vi "MS Operation.vi"(6 "PID Cluster":T3={"L1 to L4 PID Cluster"={"L1 PID Gains"={"Kp"=0.005, "Kd"=0.5, "Ki"=0.0005}, "L2 PID Gains"={"Kp"=0.01, "Kd"=1.0, "Ki"=0.005}, "L3 PID Gains"={"Kp"=0.05, "Kd"=1.0, "Ki"=0.0005}, "L4 PID Gains"={"Kp"=0.1, "Kd"=0.1, "Ki"=0.0005}}, "Stage PID Cluster"={"Stage Z PID"={"Kp"=0.0005, "Kd"=0.001, "Ki"=0.0}, "Stage Y PID"={"Kp"=0.0003, "Kd"=0.01, "Ki"=0.0}, "Stage X PID"={"Kp"=0.0003, "Kd"=0.01, "Ki"=0.0}}, "OCT Z PID Gains"={"Kp"=0.0003, "Kd"=0.0001, "Ki"=0.01}}, 8 "error in":errorcluster, 9 "Offset Home 2 RCM":dbl[](array[numeric])=[0.0, 0.0, 0.0, 0.0], 10 "Prev Posit Cluster":T2={"Prev L1 to L4 Posit"=[-0.5319, -0.035669172703475985, -2.0566170657346783, 0.9099264705882353], "Prev Stage Posit"=[6.002553885707208, 5.996566124542428, 5.995469940427586], "Prev OCT Z Posit"=-0.0}, 11 "FPGA VI Reference In":refnum<k20>) -> (0 "error out":errorcluster, 2 "Last Posit Cluster":T1={"Last L1 to L4 Posit"=[0.0, 0.0, 0.0, 0.0], "Last Stage Posit"=[6.0, 6.0, 6.0], "Last OCT Z Posit"=0.0}, 3 "FPGA VI Reference Out":refnum<k20>)   [LabVIEW 2016]
uses:
  Global Variables.vi
  <vilib>/Platform/TimedLoop/XDataNode/wakeup.ctl
  <vilib>/Platform/TimedLoop/XDataNode/XDNodeRunTimeDep.lvlib
  <vilib>/Platform/TimedLoop/XDataNode/nitl_modes.ctl
  <vilib>/Platform/TimedLoop/XDataNode/timing_clust.ctl
  <vilib>/platform/TimedLoop/XDataNode/XDataNode.xnode
  <vilib>/rvi/interface/nirviReadWriteControl/nirviReadWriteControl.xnode
  Library/KevinLibraryAll/labview/KevLib01.lvlib
  FPGA Bitfiles/PhantomControlPI_FPGATarget_QuadCtr2_E2412E44.lvbitx
  IRISS_FPGA_IO.vi
  NiFpgaLv.dll
  <vilib>/Utility/error.llb/Error Cluster From Error Code.vi
  <vilib>/rvi/errors/niLvFpgaAdjustHostInterfaceError.vi
panel:
  out "Accurus Remote cmd":T4
  out "L1 to L4 Remote cmd":sgl[](array[numeric])
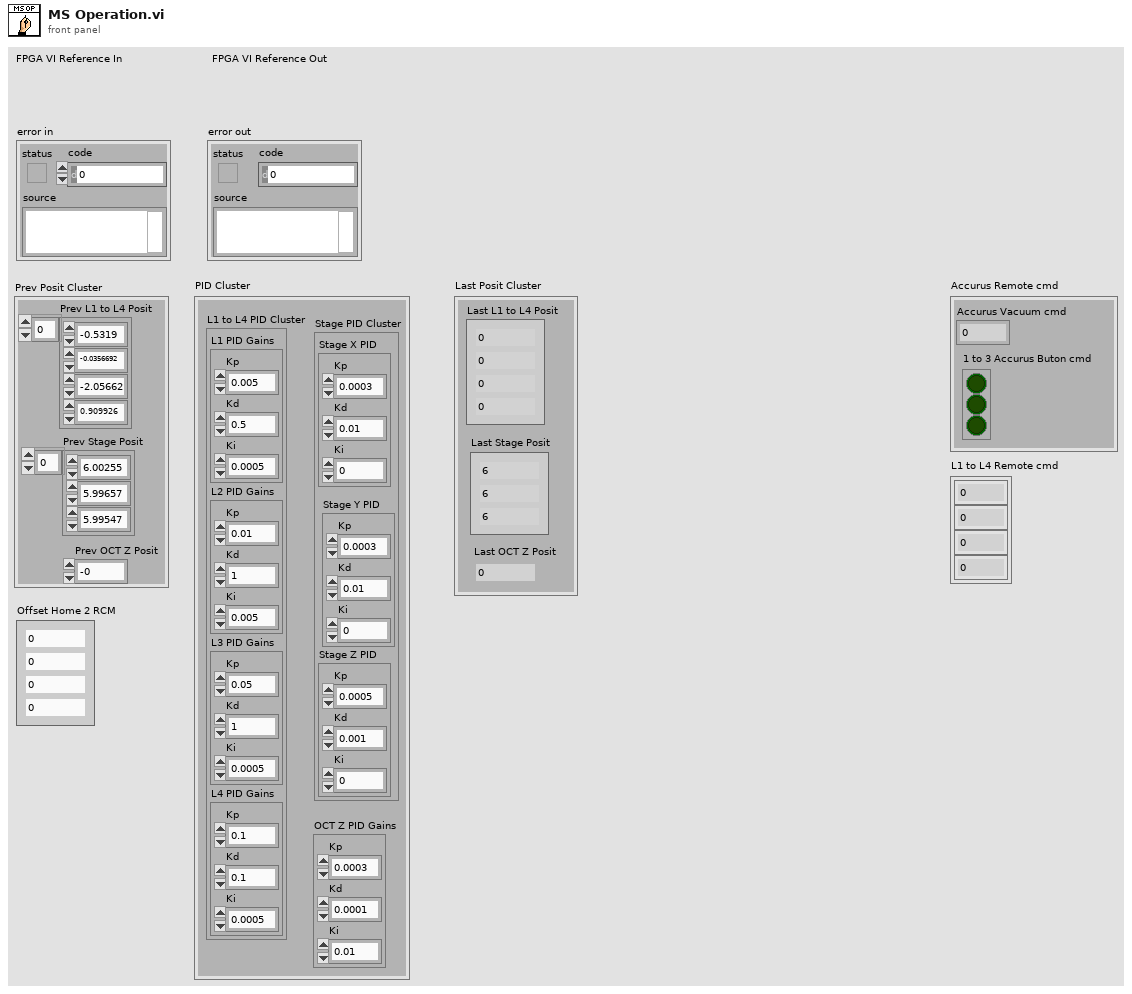
[diagram p1: front panel]
types:
  T1 = cluster{"Last L1 to L4 Posit":dbl[], "Last Stage Posit":dbl[], "Last OCT Z Posit":dbl}
  T2 = cluster{"Prev L1 to L4 Posit":dbl[], "Prev Stage Posit":dbl[], "Prev OCT Z Posit":dbl}
  T3 = cluster{"L1 to L4 PID Cluster":cluster{"L1 PID Gains":cluster{"Kp":dbl, "Kd":dbl, "Ki":dbl}, "L2 PID Gains":cluster{"Kp":dbl, "Kd":dbl, "Ki":dbl}, "L3 PID Gains":cluster{"Kp":dbl, "Kd":dbl, "Ki":dbl}, "L4 PID Gains":cluster{"Kp":dbl, "Kd":dbl, "Ki":dbl}}, "Stage PID Cluster":cluster{"Stage Z PID":cluster{"Kp":dbl, "Kd":dbl, "Ki":dbl}, "Stage Y PID":cluster{"Kp":dbl, "Kd":dbl, "Ki":dbl}, "Stage X PID":cluster{"Kp":dbl, "Kd":dbl, "Ki":dbl}}, "OCT Z PID Gains":cluster{"Kp":dbl, "Kd":dbl, "Ki":dbl}}
  T4 = cluster{"Accurus Vacuum cmd":sgl, "1 to 3 Accurus Buton cmd":bool[]}
  T5 = typedef "XDNodeRunTimeDep.lvlib/timing_clust.ctl" = cluster{"Expected End [f-1]":u64, "Actual End [f-1]":u64, "Finished Late? [f-1]":bool, "Expected End [i-1]":u64, "Actual End [i-1]":u64, "Finished Late? [i-1]":bool, "Expected Start [i]":u64, "Actual Start [i]":u64, "Expected Start [f]":u64, "Actual Start [f]":u64, "Source Name":string, "Structure Name":string, "Period":i64, "Deadline":i64, "Offset":i64, "Start":i64, "Priority":i32, "Timeout":i32, "Mode":T6, "Wakeup Reason":T7, "Error":errorcluster, "Source Type":string, "Secondary Source Type":string, "Global End Time":u64, "Global Start Time":u64, "Frame Duration":u64, "Iteration Duration":u64, "Assigned CPU":i32, "I/O Scan Engine Mode":u32}
  T6 = typedef "XDNodeRunTimeDep.lvlib/nitl_modes.ctl" = enum32{"No Change", "Process missed periods, maintain original phase", "Discard missed periods, maintain original phase", "Process missed periods, ignore original phase", "Discard missed periods, ignore original phase"}
  T7 = typedef "XDNodeRunTimeDep.lvlib/wakeup.ctl" = enum32{"Normal", "Aborted", "Asynchronous wakeup", "Timing source error", "Timed loop error", "Timeout"}
  T8 = cluster{"Stop Vacuum":bool, "Vacuum Force":i8, "Max Limit [mmHg]":dbl, "Slide in":i8, "Irrigation?":bool}
  T9 = cluster{"L1 PID Gains":cluster{"Kp":dbl, "Kd":dbl, "Ki":dbl}, "L2 PID Gains":cluster{"Kp":dbl, "Kd":dbl, "Ki":dbl}, "L3 PID Gains":cluster{"Kp":dbl, "Kd":dbl, "Ki":dbl}, "L4 PID Gains":cluster{"Kp":dbl, "Kd":dbl, "Ki":dbl}}
  T10 = cluster{"Stage Z PID":cluster{"Kp":dbl, "Kd":dbl, "Ki":dbl}, "Stage Y PID":cluster{"Kp":dbl, "Kd":dbl, "Ki":dbl}, "Stage X PID":cluster{"Kp":dbl, "Kd":dbl, "Ki":dbl}}
  T11 = cluster{"Accurus button":bool[], "Accurus engaged?":bool, "Vacuum Force":i32, "Accurus Ch. A Vout":dbl, "Accurus Ch. B Vout":dbl, "Irrigation engaged?":bool}
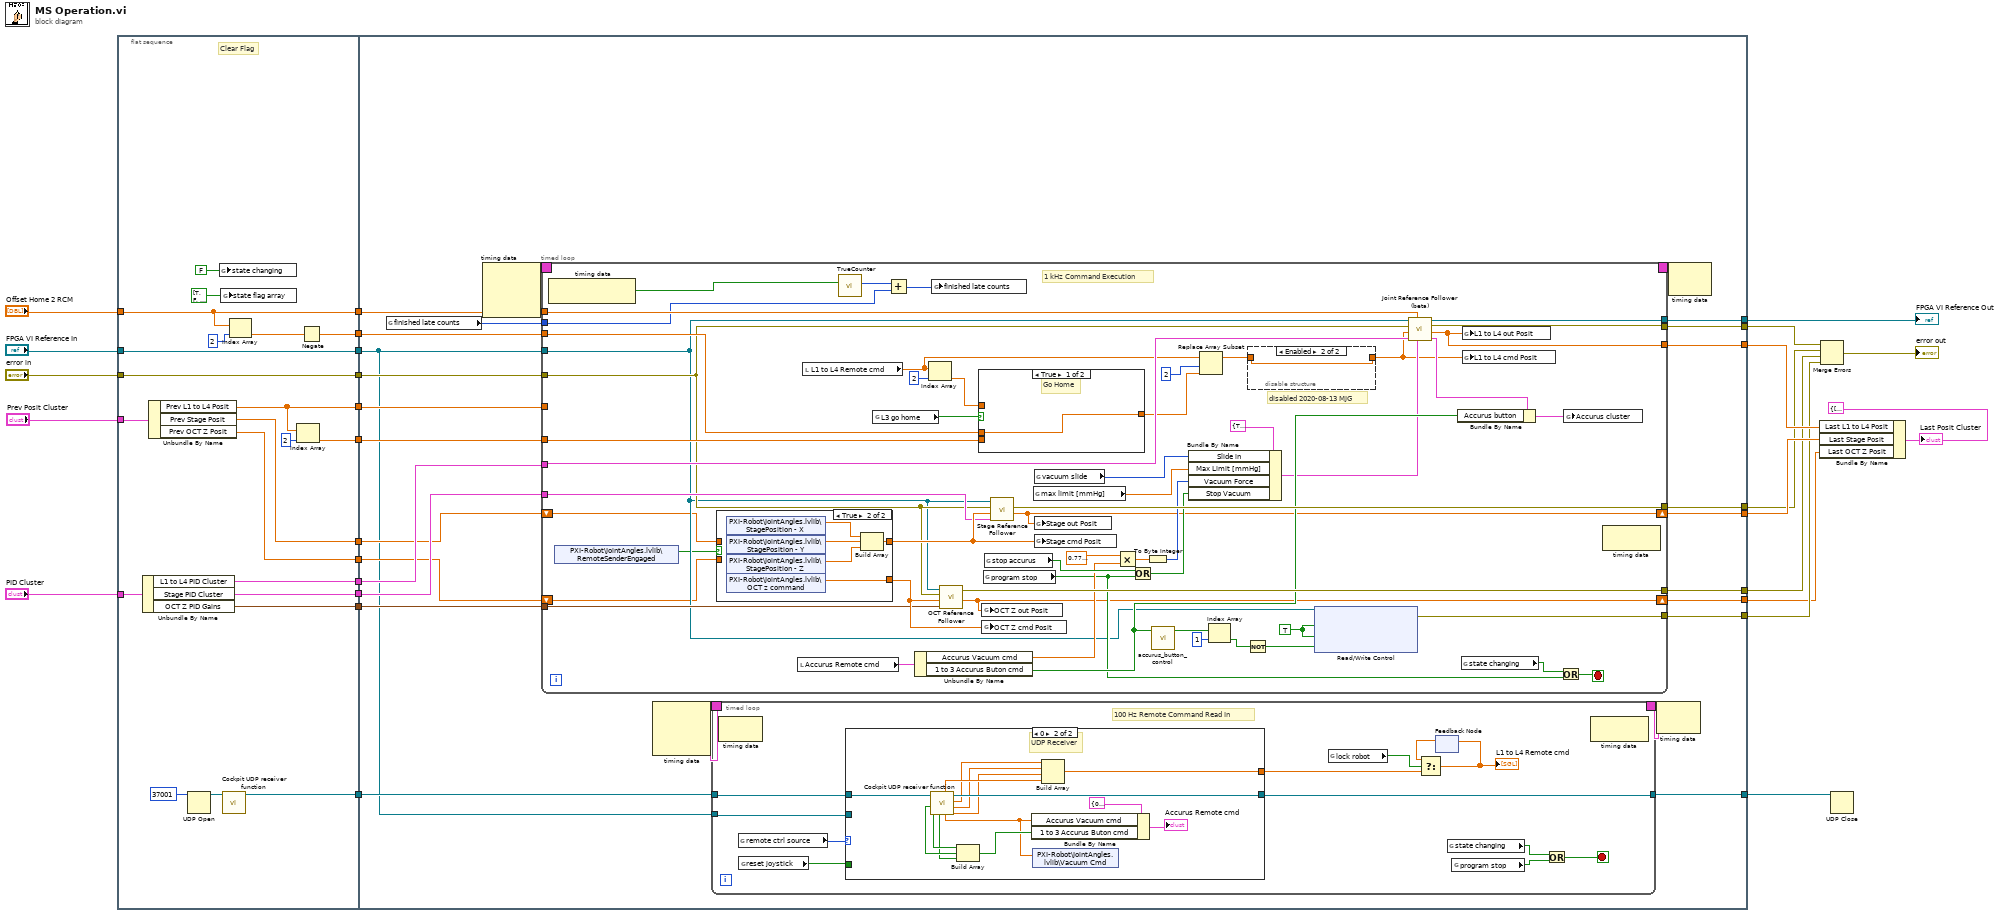
[diagram p0: block diagram]
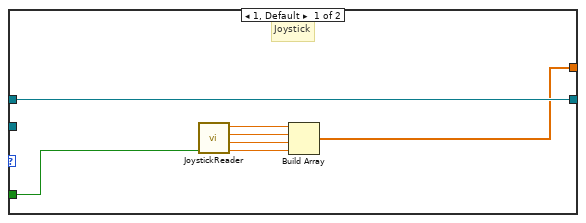
[diagram p2: hidden frame]
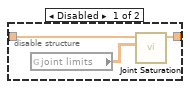
[diagram p3: hidden frame]
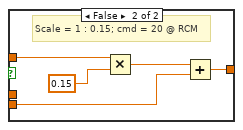
[diagram p5: hidden frame]
diagram:
  n1 = flat-sequence {
    tunnel: [w46] -> w29
    tunnel: [w45] -> w27
    tunnel: "FPGA VI Reference In" -> [w45]
    tunnel: [w44] -> w25
    tunnel: "error in" -> [w44]
    tunnel: [w37] -> w23
    tunnel: "Offset Home 2 RCM" -> [w37]
    tunnel: "Prev Posit Cluster" -> [w32]
    tunnel: [w42] -> w20
    tunnel: "PID Cluster" -> [w41]
    tunnel: [w40] -> w18
    tunnel: [w39] -> w17
    tunnel: [w35] -> w16
    tunnel: [w34] -> w4
    tunnel: [w33] -> w3
    tunnel: [w31] -> w2
    tunnel: [w30] -> w1
    tunnel: w29 -> [w72]
    tunnel: [w71] -> w28
    tunnel: w27 -> [w51]
    tunnel: w25 -> [w70]
    tunnel: w23 -> [w69]
    tunnel: w20 -> [w68]
    tunnel: w18 -> [w67]
    tunnel: w17 -> [w66]
    tunnel: w16 -> [w65]
    tunnel: [w64] -> w6
    tunnel: [w63] -> w12
    tunnel: [w62] -> w13
    tunnel: [w52] -> w10
    tunnel: [w53] -> w9
    tunnel: [w61] -> w7
    tunnel: [w60] -> w8
    tunnel: [w54] -> w5
    tunnel: w4 -> [w59]
    tunnel: w3 -> [w58]
    tunnel: w2 -> [w56]
    tunnel: w1 -> [w55]
    frame #0 {
      # "Clear Flag"
      n2 = Unbundle By Name(w41) -> ("L1 to L4 PID Cluster"=w40:T9, "Stage PID Cluster"=w34:T10, "OCT Z PID Gains"=w33:cluster{"Kp":dbl, "Kd":dbl, "Ki":dbl})
      n3 = Unbundle By Name(w32) -> ("Prev L1 to L4 Posit"=w42:dbl[], "Prev Stage Posit"=w31:dbl[], "Prev OCT Z Posit"=w30:dbl)
      n4 = UDP Open(11:u16 37001 ("port")) -> (port=w48:refnum<k16>)  [unwired: 4 in, 2 out]
      n5 = global write "Global Variables.vi" "state changing"(FALSE ("state changing")) -> ()
      n6 = global write "Global Variables.vi" "state flag array"(bool[] [TRUE, FALSE, FALSE, FALSE, FALSE, FALSE, FALSE, FALSE, FALSE] ("state flag array")) -> ()
      n7 = call "Cockpit UDP receiver function.vi"("UDP connection ID"=w48) -> ("UDP connection ID out"=w46:refnum<k16>)  [unwired: 1 in, 9 out]
      n8 = Index Array(array=w37, index=2) -> (element=w36:dbl)
      n9 = Index Array(array=w42, index=2) -> (element=w39:dbl)
      n10 = Negate(x=w36) -> (-x=w35:dbl)
    }
    frame #1 {
      n11 = global read "Global Variables.vi" "finished late counts"() -> (w57:u16)
      n12 = node-c288() -> (w76:T5)  [unwired: 3 in]
      n13 = timed-loop {
        timing: w76 -> [_]
        timing-out: [_] -> w75
        tunnel: w51 -> [w126]
        tunnel: w70 -> [w127]
        tunnel: w69 -> [w163]
        tunnel: w68 -> [_]
        tunnel: w67 -> [w160]
        tunnel: w66 -> [w159]
        tunnel: w65 -> [w156]
        tunnel: [w153] -> w64
        tunnel: [w152] -> w63
        tunnel: [w151] -> w62
        tunnel: [w150] -> w61
        tunnel: [w149] -> w60
        tunnel: w59 -> [w135]
        tunnel: w58 -> [w134]
        tunnel: w57 -> [w128]
        shift-right: [w122] -> w53
        shift-left: w56 -> [w125]
        shift-right: [w123] -> w54
        shift-left: w55 -> [w124]
        tunnel: [w119] -> w52
        stop <- w168 stop-if-true
        w147 = TRUE ("Conn0/DIO15 Button 4")
        # "disabled 2020-08-13 MJG"
        # "1 kHz Command Execution"
        n14 = node-c288() -> (w133:bool)  [unwired: 1 in]
        n15 = shared-variable "PXI-Robot\\JointAngles.lvlib\\RemoteSenderEngaged"() -> (w121:bool)  [unwired: 1 in, 1 out]
        n16 = case shown="True" w121 {
          tunnel: [w174 w179] -> w162
          tunnel: [w173 w175] -> w161
          tunnel: w125 -> [w174 _]
          tunnel: w124 -> [w173 _]
          frame False {
          }
          frame True {
            n17 = shared-variable "PXI-Robot\\JointAngles.lvlib\\StagePosition - X"() -> (w176:dbl)  [unwired: 1 in, 1 out]
            n18 = shared-variable "PXI-Robot\\JointAngles.lvlib\\StagePosition - Y"() -> (w177:dbl)  [unwired: 1 in, 1 out]
            n19 = shared-variable "PXI-Robot\\JointAngles.lvlib\\StagePosition - Z"() -> (w178:dbl)  [unwired: 1 in, 1 out]
            n20 = shared-variable "PXI-Robot\\JointAngles.lvlib\\OCT z command"() -> (w175:dbl)  [unwired: 1 in, 1 out]
            n21 = Build Array(w176, w177, w178) -> (w179:dbl[])
          }
        }
        n22 = local read "Accurus Remote cmd"() -> (w155:T4)
        n23 = local read "L1 to L4 Remote cmd"() -> (w120:sgl[])
        n24 = call "TrueCounter.vi"("True?"=w133) -> ("True Count"=w129:u16)  [unwired: 10 in]
        n25 = global read "Global Variables.vi" "L3 go home"() -> (w166:bool)
        n26 = Add(x=w129, y=w128) -> (x+y=w130:u16)
        n27 = Unbundle By Name(w155) -> ("Accurus Vacuum cmd"=w140:sgl, "1 to 3 Accurus Buton cmd"=w142:bool[])
        n28 = Index Array(array=w120, index=2) -> (element=w164:sgl)
        n29 = global write "Global Variables.vi" "finished late counts"(w130) -> ()
        n30 = call "OCT Reference Follower.vi"("OCT Z PID Gains"=w134, "OCT  Z cmd Posit [mm]"=w161, "error in"=w127, "FPGA VI Reference In"=w126) -> ("OCT  Z out Posit [mm]"=w123:dbl, "error out"=w150:errorcluster)  [unwired: 5 in, 1 out]
        n31 = case shown="True" w166 {
          tunnel: [w180 w185] -> w157
          tunnel: w164 -> [_ w182]
          tunnel: w159 -> [_ w181]
          tunnel: w156 -> [w180 _]
          frame True {
            # "Go Home"
          }
          frame False {
            # "Scale = 1 : 0.15; cmd = 20 @ RCM"
            n32 = Multiply(x=w182, y=0.15) -> (x*y=w184:dbl)
            n33 = Add(x=w184, y=w181) -> (x+y=w185:dbl)
          }
        }
        n34 = global write "Global Variables.vi" "OCT Z out Posit"(w123) -> ()
        n35 = global write "Global Variables.vi" "OCT Z cmd Posit"(w161) -> ()
        n36 = global read "Global Variables.vi" "program stop"() -> (w138:bool)
        n37 = global read "Global Variables.vi" "stop accurus"() -> (w141:bool)
        n38 = call "Stage Reference Follower.vi"("Stage PID Cluster"=w135, "Stage cmd Posit [mm]"=w162, "error in"=w127, "FPGA VI Reference In"=w126) -> ("Stage out Posit [mm]"=w122:dbl[], "error out"=w149:errorcluster)  [unwired: 5 in, 1 out]
        n39 = global read "Global Variables.vi" "max limit [mmHg]"() -> (w131:dbl)
        n40 = global read "Global Variables.vi" "vacuum slide"() -> (w132:i8)
        n41 = global write "Global Variables.vi" "Stage out Posit"(w122) -> ()
        n42 = global write "Global Variables.vi" "Stage cmd Posit"(w162) -> ()
        n43 = Multiply(x=sgl 0.78 ("y"), y=w140) -> (x*y=w154:sgl)
        n44 = Or(x=w141, y=w138) -> (x .or. y?=w137:bool)
        n45 = To Byte Integer(number=w154) -> (8bit integer=w136:i8)
        n46 = call "accurus_button_control.vi"("Array in"=w142) -> ("Array out"=w146:bool[])  [unwired: 10 in]
        n47 = Bundle By Name(cluster=T8 {"Stop Vacuum"=TRUE, "Vacuum Force"=0, "Max Limit [mmHg]"=600.0, "Slide in"=0, "Irrigation?"=FALSE} ("Accurus Ctrl Cluster"), "Slide in"=w132, "Max Limit [mmHg]"=w131, "Vacuum Force"=w136, "Stop Vacuum"=w137) -> (w117:T8)
        n48 = Replace Array Subset(array=w120, new element=w157, index=2) -> (w114:sgl[])
        n49 = Index Array(array=w146, index=1) -> (element=w145:bool)
        n50 = Not(x=w145) -> (.not. x?=w144:bool)
        n51 = disable-structure shown="Enabled" {
          disable-tunnel: [w171 w172] -> w115
          disable-tunnel: w114 -> [w170 w172]
          frame Disabled {
            n52 = global read "Global Variables.vi" "joint limits"() -> (w169:dbl[][])
            n53 = call "Joint Saturation.vi"("Joint Bounds [Deg/mm]"=w169, "Ref Array [Deg/mm]"=w170) -> ("Sat Ref Array [Deg/mm]"=w171:dbl[])  [unwired: 9 in]
          }
          frame Enabled {
          }
        }
        n54 = xnode "Read/Write Control"("FPGA VI Reference In"=w126, "Conn0/DIO12 Button 1"=w147, "Conn0/DIO13 Button 2"=w147, "Conn0/DIO15 Button 4"=w144) -> ("error out"=w153:errorcluster)  [unwired: 1 in, 1 out]
        n55 = call "Joint Reference Follower (beta).vi"("Accurus Ctrl Cluster"=w117, "Offset Home2RCM [deg/mm]"=w163, "PID Ctrl Cluster"=w160, "Ref Array [deg/mm]"=w115, "error in"=w127, "FPGA VI Reference In"=w126) -> ("Accurus Output Cluster"=w116:T11, "Output Posit Array [deg/mm]"=w119:dbl[], "error out"=w152:errorcluster, "FPGA VI Reference Out"=w151:refnum<k20>)  [unwired: 2 in]
        n56 = Bundle By Name(cluster=w116, "Accurus button"=w142) -> (w143:T11)
        n57 = global read "Global Variables.vi" "state changing"() -> (w167:bool)
        n58 = global write "Global Variables.vi" "L1 to L4 out Posit"(w119) -> ()
        n59 = global write "Global Variables.vi" "L1 to L4 cmd Posit"(w115) -> ()
        n60 = Or(x=w167, y=w138) -> (x .or. y?=w168:bool)
        n61 = global write "Global Variables.vi" "Accurus cluster"(w143) -> ()
        n62 = node-c288() -> ()  [unwired: 1 in, 1 out]
      }
      n63 = node-c288() -> (w74:T5)  [unwired: 3 in]
      n64 = timed-loop {
        timing: w74 -> [_]
        timing-out: [_] -> w73
        tunnel: w72 -> [w85]
        tunnel: [w84] -> w71
        tunnel: w51 -> [w83]
        stop <- w88 stop-if-true
        # "100 Hz Remote Command Read In"
        n65 = node-c288() -> ()  [unwired: 1 in, 1 out]
        n66 = global read "Global Variables.vi" "remote ctrl source"() -> (w82:u16)
        n67 = global read "Global Variables.vi" "reset joystick"() -> (w81:bool)
        n68 = case shown="0" w82 {
          tunnel: [w94 w109] -> w84
          tunnel: w85 -> [w94 w98]
          tunnel: w81 -> [w95 _]
          tunnel: w83 -> [_ _]
          tunnel: [w89 w97] -> w77
          frame 1, Default {
            # "Joystick"
            n69 = call "JoystickReader.vi"("Reset"=w95) -> ("L4 [deg]"=w90:sgl, "L3 [0~100]"=w91:sgl, "L2 [deg]"=w92:sgl, "L1 [deg]"=w93:sgl)  [unwired: 7 in]
            n70 = Build Array(w93, w92, w91, w90) -> (w89:sgl[])
          }
          frame 0 {
            # "UDP Receiver"
            n71 = call "Cockpit UDP receiver function.vi"("UDP connection ID"=w98) -> ("L3"=w106:sgl, "L2"=w105:sgl, "L1"=w107:sgl, "UDP connection ID out"=w109:refnum<k16>, "down_pedal"=w96:sgl, "L4"=w108:sgl, "right_pedal"=w100:bool, "left_pedal"=w102:bool, "up_pedal"=w101:bool)  [unwired: 1 in, 1 out]
            n72 = Build Array(w102, w101, w100) -> (w99:bool[])
            n73 = Bundle By Name(cluster=T4 {"Accurus Vacuum cmd"=0.0, "1 to 3 Accurus Buton cmd"=[FALSE, FALSE, FALSE]} ("Accurus Cockpit cmd 2"), "Accurus Vacuum cmd"=w96, "1 to 3 Accurus Buton cmd"=w99) -> (→"Accurus Remote cmd":T4)
            n74 = shared-variable "PXI-Robot\\JointAngles.lvlib\\Vacuum Cmd"(w96) -> ()  [unwired: 1 in, 1 out]
            n75 = Build Array(w107, w105, w106, w108) -> (w97:sgl[])
          }
        }
        n76 = global read "Global Variables.vi" "lock robot"() -> (w80:bool)
        n77 = feedback #1() -> (w79:sgl[])  [unwired: 1 in]
        n78 = Select(t=w79, s=w80, f=w77) -> (s? t:f=w78:sgl[])
        "L1 to L4 Remote cmd" <- w78
        n79 = feedback-in #1(w78) -> ()
        n80 = global read "Global Variables.vi" "state changing"() -> (w87:bool)
        n81 = global read "Global Variables.vi" "program stop"() -> (w86:bool)
        n82 = Or(x=w87, y=w86) -> (x .or. y?=w88:bool)
        n83 = node-c288() -> ()  [unwired: 1 in, 1 out]
      }
      n84 = node-c288(w73) -> ()  [unwired: 1 out]
      n85 = node-c288(w75) -> ()  [unwired: 1 out]
    }
  }
  n86 = Bundle By Name(cluster=T1 {"Last L1 to L4 Posit"=[-0.5607, -0.038216970753724266, -2.0806193533568895, 1.1787683823529411], "Last Stage Posit"=[6.002553885707208, 5.996566124542428, 5.995469940427586], "Last OCT Z Posit"=-0.0} ("Last Posit Cluster 2"), "Last L1 to L4 Posit"=w10, "Last Stage Posit"=w9, "Last OCT Z Posit"=w5) -> (→"Last Posit Cluster":T1)
  n87 = Merge Errors(w12, w8, w7, w6) -> (→"error out":errorcluster)
  n88 = UDP Close(connection ID=w28) -> ()  [unwired: 1 in, 2 out]
  "FPGA VI Reference Out" <- w13
